vi "svc_Set dB ref if Pascal.vi"(4 "channel info":T1={"sensor sensitivity"=1000.0, "engineering units"=1, "dB reference"=1.0, "custom label"="EU", "weighting filter"=0, "pregain"=0.0} {"pregain" format="%.2f"; "weighting filter" items=["Linear", "A-weighting", "B-weighting", "C-weighting", "ITU-R 468-4", "Dolby", "CCITT", "C-message", "Wb", "Wc", "Wd", "We", "Wf", "Wh", "Wj", "Wk", "Wm", "AES17 20 kHz lowpass", "AES17 40 kHz lowpass", "AES17 20 kHz highpass", "AES17 40 kHz highpass"]; "dB reference" format="%^.1e"; "engineering units" items=["custom..."=0, "V"=1, "A"=21, "C"=30, "pC"=31, "s"=32, "-"=29, "Pa"=2, "N"=20, "g"=3, "m/s^2"=4, "m/s"=5, "m"=6, "mm/s"=12, "mm"=13, "micron/s"=14, "micron"=15, "in/s^2"=7, "in/s"=8, "in"=9, "mil/s"=10, "mil"=11, "rad/s^2"=16, "rad/s"=17, "rad"=18, "deg/s^2"=26, "deg/s"=27, "deg"=28, "RPM"=22, "cycle/s^2"=23, "Hz"=24, "cycle"=25, "strain"=19]; "sensor sensitivity" format="%#_5f"}, 7 "unit label":string) -> (0 "channel info":T1={"sensor sensitivity"=1000.0, "engineering units"=1, "dB reference"=1.0, "custom label"="EU", "weighting filter"=0, "pregain"=0.0} {"pregain" format="%.2f"; "weighting filter" items=["Linear", "A-weighting", "B-weighting", "C-weighting", "ITU-R 468-4", "Dolby", "CCITT", "C-message", "Wb", "Wc", "Wd", "We", "Wf", "Wh", "Wj", "Wk", "Wm", "AES17 20 kHz lowpass", "AES17 40 kHz lowpass", "AES17 20 kHz highpass", "AES17 40 kHz highpass"]; "dB reference" format="%^.1e"; "engineering units" items=["custom..."=0, "V"=1, "A"=21, "C"=30, "pC"=31, "s"=32, "-"=29, "Pa"=2, "N"=20, "g"=3, "m/s^2"=4, "m/s"=5, "m"=6, "mm/s"=12, "mm"=13, "micron/s"=14, "micron"=15, "in/s^2"=7, "in/s"=8, "in"=9, "mil/s"=10, "mil"=11, "rad/s^2"=16, "rad/s"=17, "rad"=18, "deg/s^2"=26, "deg/s"=27, "deg"=28, "RPM"=22, "cycle/s^2"=23, "Hz"=24, "cycle"=25, "strain"=19]; "sensor sensitivity" format="%#_5f"}, 3 "dup unit label":string)   [LabVIEW 2017]
uses:
  <vilib>/addons/_NISVFA/_Shared subVIs/Controls/svc_Channel Info.ctl
  <vilib>/addons/_NISVFA/_Shared subVIs/Controls/svc_Engineering Units Text Ring.ctl
  <vilib>/addons/_NISVFA/_Shared subVIs/Controls/svc_Weighting Filter Text Ring.ctl
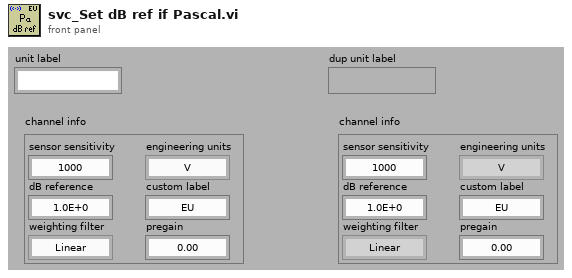
[diagram p1: front panel]
types:
  T1 = typedef "svc_Channel Info.ctl" = cluster{"sensor sensitivity":dbl, "engineering units":T2, "dB reference":dbl, "custom label":string, "weighting filter":T3, "pregain":dbl}
  T2 = typedef "svc_Engineering Units Text Ring.ctl" = u16
  T3 = typedef "svc_Weighting Filter Text Ring.ctl" = u16
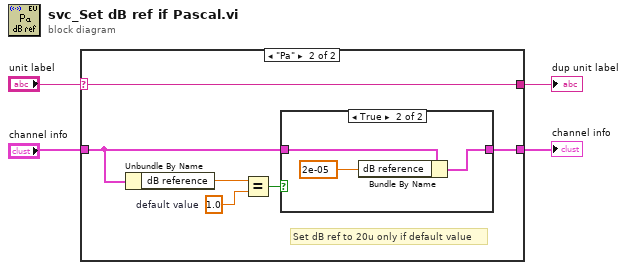
[diagram p0: block diagram]
diagram:
  n1 = case shown="\"Pa\"" "unit label" {
    selector: "unit label" -> [w5 w12]
    tunnel: "channel info" -> [w6 w10]
    tunnel: [w6 w11] -> w2
    tunnel: [w5 w12] -> w1
    frame Default {
    }
    frame "Pa" {
      w8 = 1.0  # default value
      # "Set dB ref to 20u only if default value"
      n2 = Unbundle By Name(w10) -> ("dB reference"=w9:dbl)
      n3 = Equal?(x=w9, y=w8) -> (x = y?=w7:bool)
      n4 = case shown="True" w7 {
        tunnel: [w13 w15] -> w11
        tunnel: w10 -> [w13 w14]
        frame False {
        }
        frame True {
          n5 = Bundle By Name(cluster=w14, "dB reference"=2e-05 ("dB reference [EU]")) -> (w15:T1)
        }
      }
    }
  }
  "channel info" <- w2
  "dup unit label" <- w1
